vi "BITalino.vi"() -> ()   [LabVIEW 2015]
uses:
  Status.ctl
  Sensor.ctl
  <vilib>/Instr/_visa.llb/VISA Configure Serial Port (Instr).vi
panel:
  in  "DO 4":bool
  in  "DO 3":bool
  in  "DO 2":bool
  in  "DO 1":bool
  in  "Battery \nThreshold (%)":u8(slide)=5 min=5 max=90 step=5 scale=5.0..90.0
  out "CRC Error":bool
  out "tdms file":refnum<k34>
  out "XY Graph":cluster{dbl[], dbl[]}(graph)
  out "Ylabel and Plot name":cluster{string, string}
  out "Sample Rate Numeric":i32
  out "Consumer":i32
  out "producer":i32
  in  "Sensor Selection":enum32{"A1", "A2", "A3", "A4", "A5", "A6"}(radio)
  in  "Sensor 6":T1=enum."LUX"
  in  "Sensor 5":T1=enum."ACC"
  in  "Sensor 4":T1=enum."EDA"
  in  "Sensor 3":T1=enum."EEG"
  in  "Sensor 2":T1=enum."ECG"
  in  "Sensor 1":T1
  out "DI 2":bool
  out "DI 1":bool
  out "DI 4":bool
  out "DI 3":bool
  in  "MODE":bool
  in  "Sample Rate":enum16{"1", "10", "100", "1000"}(ring)=enum."1000"
  in  "error in (no error)":errorcluster
  in  "File Path":path
  in  "X Limit":u32(knob)=5 scale=2.0..30.0
  in  "Device":refnum<visa-resource-name>
  out "Sync Stop":bool=TRUE
  out "Status":T2
  in  "Exit Button":bool
  in  "Record Button":bool
  in  "Stop Button":bool
  # "LIVE MODE"
  # "SIMULATED MODE"
  # "Hz"
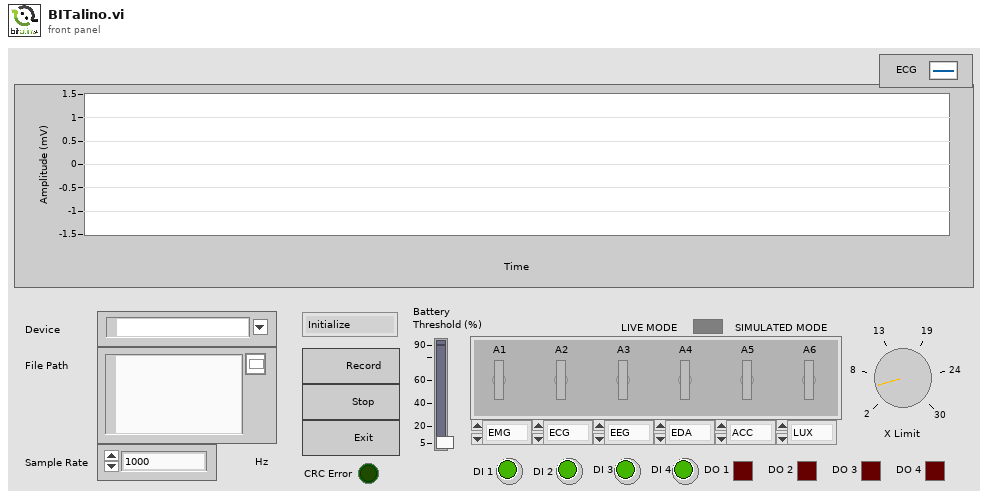
[diagram p1: front panel]
types:
  T1 = typedef "Sensor.ctl" = enum16{"EMG", "ECG", "EEG", "EDA", "ACC", "LUX"}
  T2 = typedef "Status.ctl" = enum16{"Initialize", "Standby", "Recording", "Exit"}
  T3 = enum8{"Enabled", "Disabled", "Disabled and Grayed Out"}
  T4 = enum16{"open", "open or create", "create or replace", "create", "open (read-only)"}
  T5 = cluster{"Sensor 1":T1, "Sensor 2":T1, "Sensor 3":T1, "Sensor 4":T1, "Sensor 5":T1, "Sensor 6":T1}
  T6 = cluster{"Result":dbl, "Result":dbl, "Result":dbl, "Result":dbl, "Result":dbl, "Result":dbl}
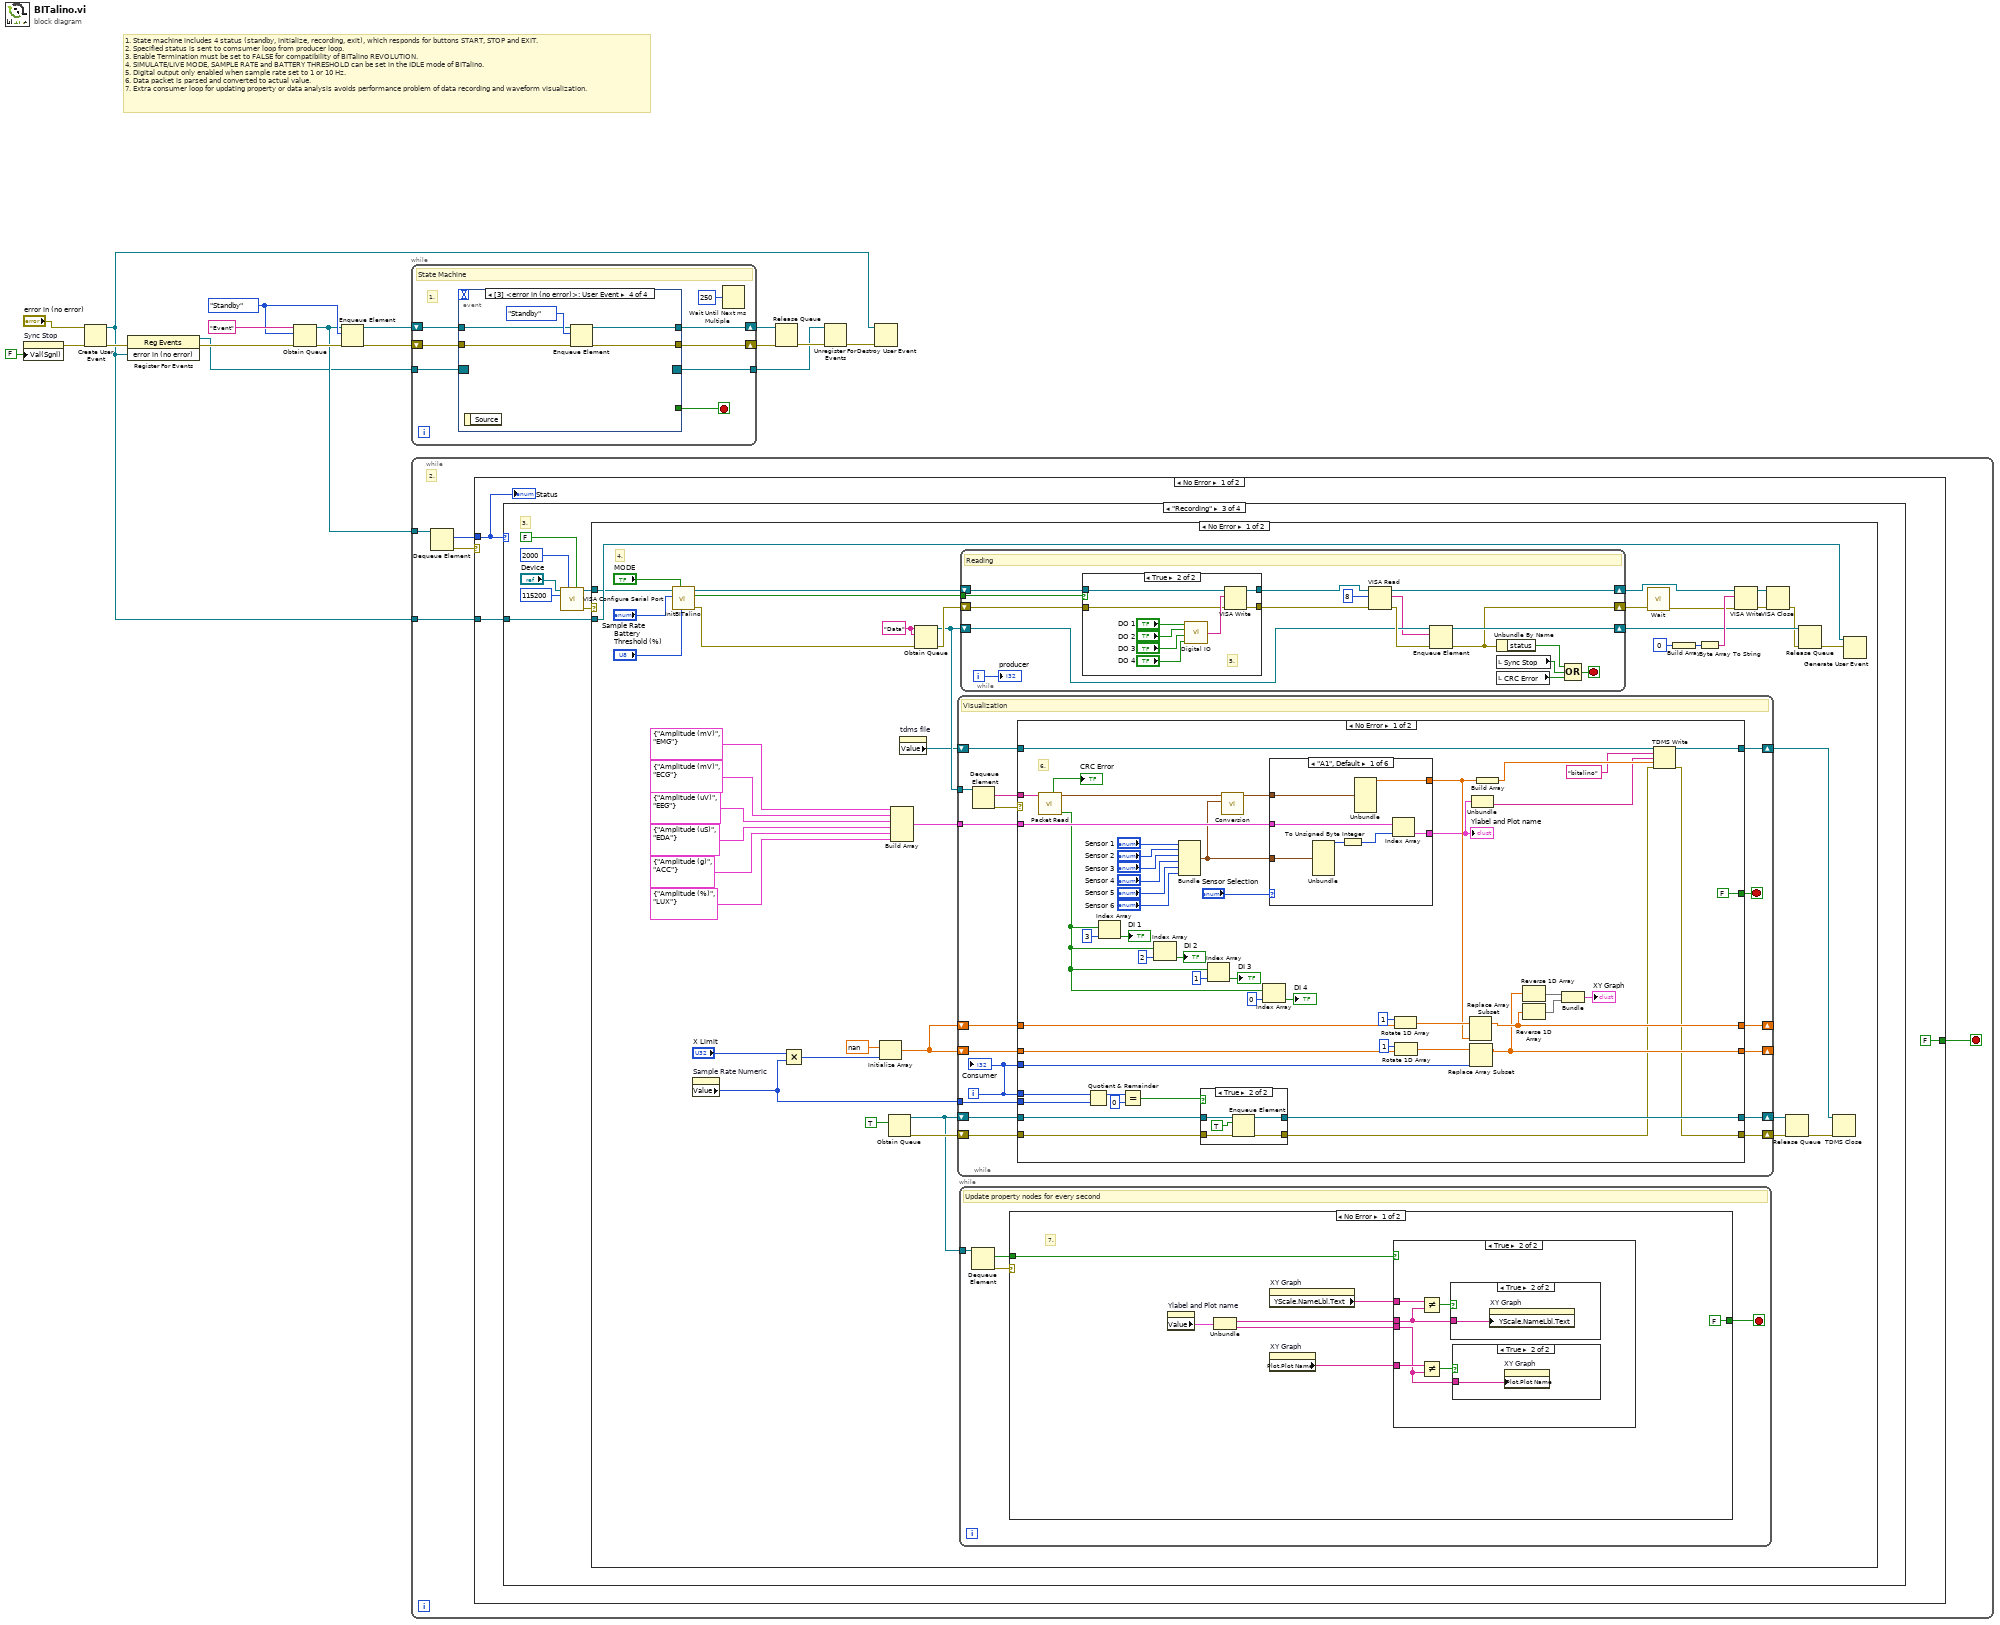
[diagram p0: block diagram]
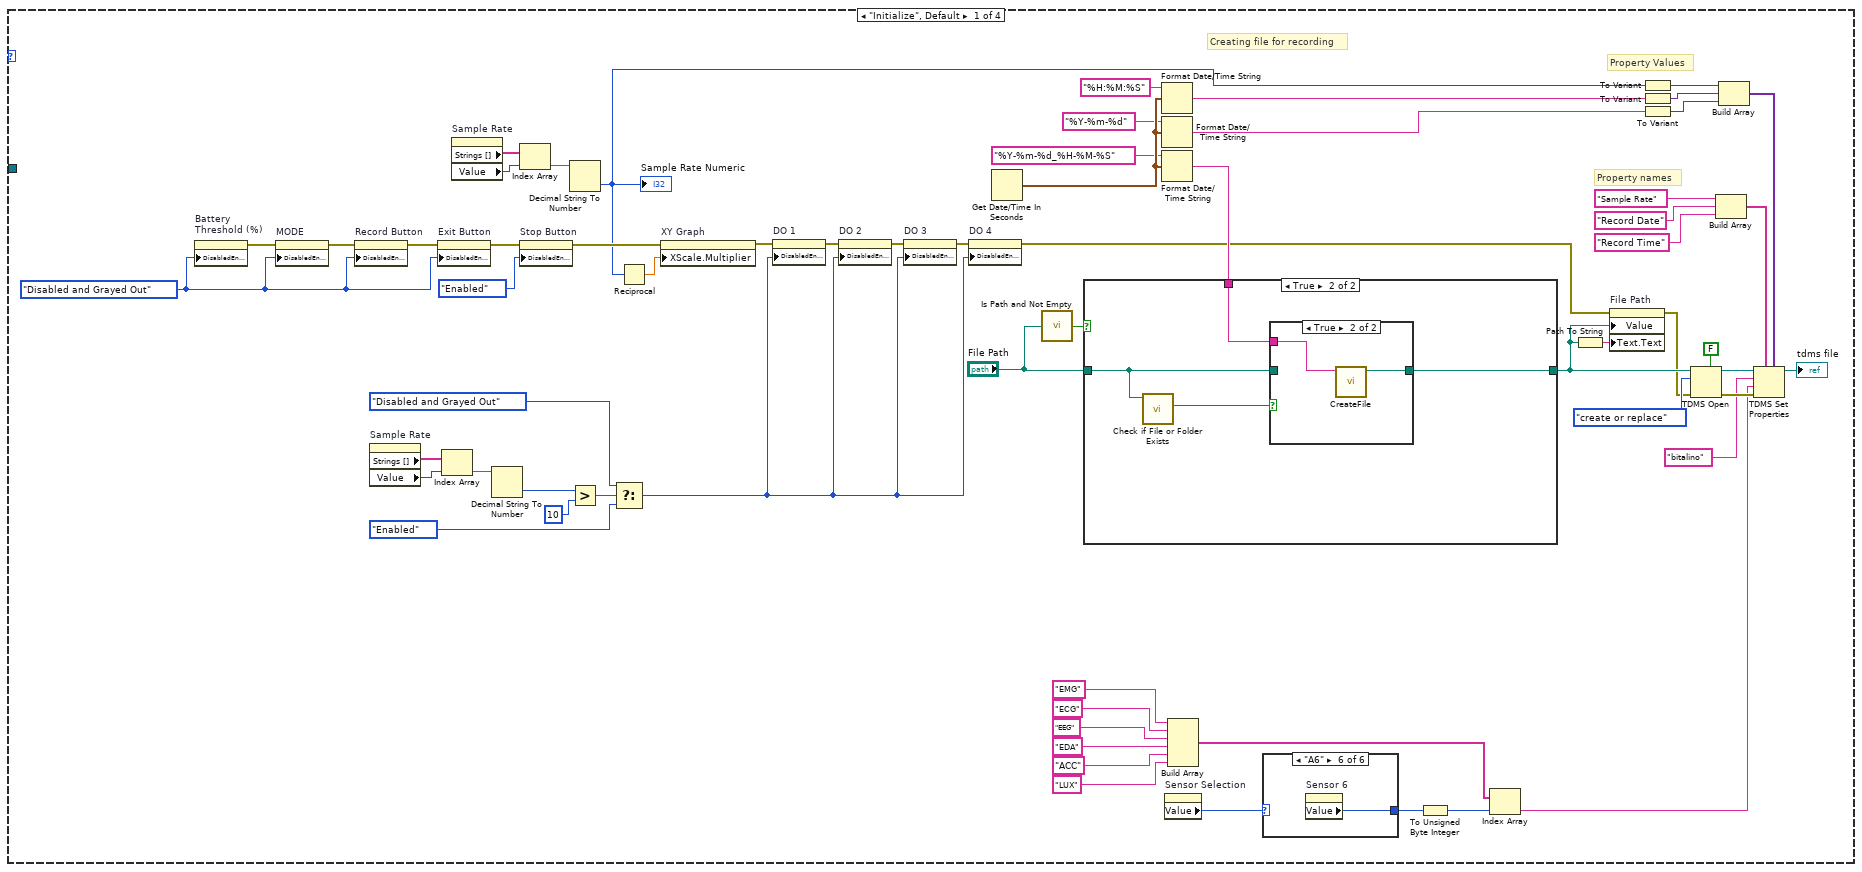
[diagram p2: hidden frame]
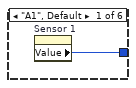
[diagram p3: hidden frame]
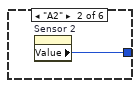
[diagram p4: hidden frame]
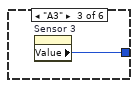
[diagram p5: hidden frame]
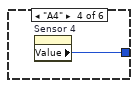
[diagram p6: hidden frame]
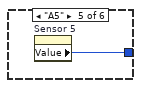
[diagram p7: hidden frame]
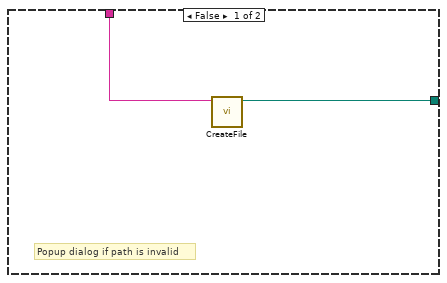
[diagram p8: hidden frame]
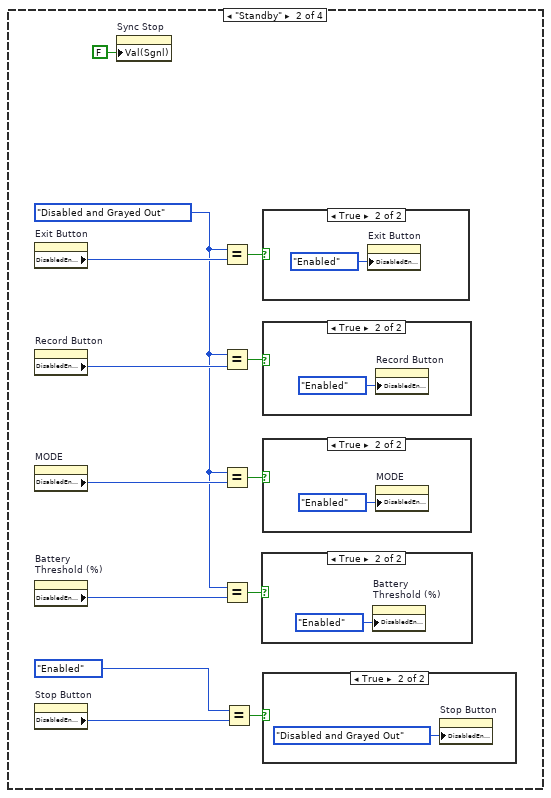
[diagram p10: hidden frame]
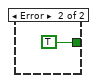
[diagram p19: hidden frame]
diagram:
  w12 = Status."Standby" ("Enum")
  # "1. State machine includes 4 status (standby, initialize, recording, exit), which responds for buttons START, STOP and EXIT.\n2. Specified status is sent to comsumer loop from producer loop.\n3. Enable Termination must be set to FALSE for compatibility of BITalino REVOLUTION.\n4. SIMULATE/LIVE MODE, SAMPLE RATE and BATTERY THRESHOLD can be set in the IDLE mode of BITalino.\n5. Digital output only enabled when sample rate set to 1 or 10 Hz.\n6. Data packet is parsed and converted to actual value.\n7. Extra consumer loop for updating property or data analysis avoids performance problem of data recording and waveform visualization."
  n1 = property on="Sync Stop" class="Bool (strict)"("Val(Sgnl)"=FALSE ("Value (Signaling)")) -> (error out=w9:errorcluster)  [unwired: 2 in, 1 out]
  n2 = Create User Event(user event datatype="error in (no error)", error in=w9) -> (user event=w1:refnum<user-event>, error out=w8:errorcluster)
  n3 = register-events(error in=w8, w1) -> (reference out=w6:refnum<event-registration>, error out=w7:errorcluster)  [unwired: 1 in]
  n4 = Obtain Queue(name (unnamed)="Event", element data type=w12, error in (no error)=w7) -> (queue out=w11:refnum<queue>, error out=w15:errorcluster)  [unwired: 2 in, 1 out]
  n5 = Enqueue Element(queue=w11, element=w12, error in (no error)=w15) -> (queue out=w13:refnum<queue>, error out=w14:errorcluster)  [unwired: 1 in, 1 out]
  n6 = while {
    shift-right: [w23] -> w17
    shift-left: w13 -> [w26]
    shift-right: [w24] -> w16
    shift-left: w14 -> [w25]
    tunnel: w6 -> [w20]
    tunnel: [w19] -> w3
    stop <- w22 stop-if-true
    # "1."
    # "State Machine"
    n7 = event shown="[3] <error in (no error)>: User Event" {
      selector: w20 -> [_ _ _ _]
      dyn-events: [_ _ _ _] -> w19
      timeout: _ -> [_ _ _ _]
      tunnel: w26 -> [w33 w37 w49 w53]
      tunnel: w25 -> [w30 w39 w48 w51]
      tunnel: [w27 w40 w43 w50] -> w24
      tunnel: [w34 w38 w45 w52] -> w23
      tunnel: [FALSE TRUE FALSE _] -> w22
      event "Stop Button": Value Change {
        n8 = event-data() -> ()  [unwired: 1 in, 5 out]
        n9 = Enqueue Element(queue=w33, element=Status."Standby" ("Enum"), error in (no error)=w30) -> (queue out=w34:refnum<queue>, error out=w28:errorcluster)  [unwired: 1 in, 1 out]
        n10 = property on="Sync Stop" class="Bool (strict)"(error in=w28, "Val(Sgnl)"=TRUE) -> (error out=w27:errorcluster)  [unwired: 1 in, 1 out]
      }
      event "Exit Button": Value Change {
        n11 = event-data() -> ()  [unwired: 1 in, 5 out]
        n12 = Enqueue Element(queue=w37, element=Status."Exit" ("Enum"), error in (no error)=w39) -> (queue out=w38:refnum<queue>, error out=w40:errorcluster)  [unwired: 1 in, 1 out]
      }
      event "Record Button": Value Change {
        n13 = event-data() -> ()  [unwired: 1 in, 1 out]
        n14 = Enqueue Element(queue=w49, element=Status."Initialize" ("Enum"), error in (no error)=w48) -> (queue out=w46:refnum<queue>, error out=w44:errorcluster)  [unwired: 1 in, 1 out]
        n15 = Enqueue Element(queue=w46, element=Status."Recording" ("Enum"), error in (no error)=w44) -> (queue out=w45:refnum<queue>, error out=w43:errorcluster)  [unwired: 1 in, 1 out]
      }
      event User Event {
        n16 = event-data() -> ()  [unwired: 1 in, 1 out]
        n17 = Enqueue Element(queue=w53, element=Status."Standby" ("Enum"), error in (no error)=w51) -> (queue out=w52:refnum<queue>, error out=w50:errorcluster)  [unwired: 1 in, 1 out]
      }
    }
    n18 = Wait Until Next ms Multiple(millisecond multiple=u32 250) -> ()  [unwired: 1 out]
  }
  n19 = while {
    tunnel: w11 -> [w58]
    tunnel: w1 -> [w55]
    stop <- w59 stop-if-true
    # "2."
    n20 = Dequeue Element(queue=w58) -> (element=w57:T2, error out=w56:errorcluster)  [unwired: 2 in, 2 out]
    n21 = case shown="No Error" w56 {
      tunnel: w57 -> [w61 _]
      tunnel: [FALSE TRUE] -> w59
      tunnel: w55 -> [w60 _]
      frame No Error {
        n22 = case shown="\"Recording\"" w61 {
          tunnel: w60 -> [_ _ w159 _]
          frame "Initialize", Default {
            w90 = T3."Disabled and Grayed Out" ("Disabled")
            # "Creating file for recording"
            # "Property Values"
            # "Property names"
            n23 = property on="Battery \nThreshold (%)" class="Slide (strict)"("DisabledEnum"=w90) -> (error out=w91:errorcluster)  [unwired: 2 in, 1 out]
            n24 = property on="MODE" class="Bool (strict)"(error in=w91, "DisabledEnum"=w90) -> (error out=w117:errorcluster)  [unwired: 1 in, 1 out]
            n25 = property on="Record Button" class="Bool"(error in=w117, "DisabledEnum"=w90) -> (error out=w125:errorcluster)  [unwired: 1 in, 1 out]
            n26 = property on="Sample Rate" class="Enum (strict)"() -> ("Strings []"=w80:string[], "Value"=w79:enum16{"1", "10", "100", "1000"})  [unwired: 2 in, 2 out]
            n27 = property on="Exit Button" class="Bool"(error in=w125, "DisabledEnum"=w90) -> (error out=w123:errorcluster)  [unwired: 1 in, 1 out]
            n28 = Index Array(array=w80, index=w79) -> (element=w78:string)
            n29 = property on="Sample Rate" class="Enum (strict)"() -> ("Strings []"=w122:string[], "Value"=w121:enum16{"1", "10", "100", "1000"})  [unwired: 2 in, 2 out]
            n30 = Decimal String To Number(string=w78) -> (number=w77:i32)  [unwired: 2 in, 1 out]
            n31 = Index Array(array=w122, index=w121) -> (element=w120:string)
            n32 = property on="Stop Button" class="Bool"(error in=w123, "DisabledEnum"=T3."Enabled" ("Disabled")) -> (error out=w119:errorcluster)  [unwired: 1 in, 1 out]
            n33 = Decimal String To Number(string=w120) -> (number=w89:i32)  [unwired: 2 in, 1 out]
            "Sample Rate Numeric" <- w89
            n34 = Greater?(x=w77, y=10) -> (0:w85:bool)
            n35 = Select(t=T3."Disabled and Grayed Out" ("Disabled"), s=w85, f=T3."Enabled" ("Disabled")) -> (s? t:f=w88:T3)
            n36 = Reciprocal(x=w89) -> (1/x=w118:dbl)
            n37 = property on="XY Graph" class="XYGraph (strict)"(error in=w119, "XScale.Multiplier"=w118) -> (error out=w76:errorcluster)  [unwired: 1 in, 1 out]
            n38 = property on="DO 1" class="Bool (strict)"(error in=w76, "DisabledEnum"=w88) -> (error out=w83:errorcluster)  [unwired: 1 in, 1 out]
            n39 = property on="DO 2" class="Bool (strict)"(error in=w83, "DisabledEnum"=w88) -> (error out=w82:errorcluster)  [unwired: 1 in, 1 out]
            n40 = property on="DO 3" class="Bool (strict)"(error in=w82, "DisabledEnum"=w88) -> (error out=w81:errorcluster)  [unwired: 1 in, 1 out]
            n41 = property on="DO 4" class="Bool (strict)"(error in=w81, "DisabledEnum"=w88) -> (error out=w75:errorcluster)  [unwired: 1 in, 1 out]
            n42 = Get Date/Time In Seconds() -> (seconds since 1Jan1904=w107:timestamp)
            n43 = call <vilib>:"Is Path and Not Empty.vi"("path"="File Path") -> ("Is Path and Not Empty?"=w99:bool)  [unwired: 4 in]
            n44 = Format Date/Time String(time format string (%c)="%H:%M:%S", seconds (now)=w107) -> (date/time string=w112:string)  [unwired: 1 in]
            n45 = Format Date/Time String(time format string (%c)="%Y-%m-%d", seconds (now)=w107) -> (date/time string=w113:string)  [unwired: 1 in]
            n46 = Format Date/Time String(time format string (%c)="%Y-%m-%d_%H-%M-%S", seconds (now)=w107) -> (date/time string=w103:string)  [unwired: 1 in]
            n47 = case shown="True" w99 {
              tunnel: [w132 w135] -> w96
              tunnel: "File Path" -> [_ w134]
              tunnel: w103 -> [w133 w136]
              frame False {
                # "Popup dialog if path is invalid"
                n48 = call "CreateFile.vi"("date/time string"=w133) -> ("appended path"=w132:path)  [unwired: 10 in]
              }
              frame True {
                n49 = call <vilib>:"Check if File or Folder Exists.vi"("path"=w134) -> ("file or folder exists?"=w137:bool)  [unwired: 8 in, 2 out]
                n50 = case shown="True" w137 {
                  tunnel: w136 -> [_ w140]
                  tunnel: [w138 w139] -> w135
                  tunnel: w134 -> [w138 _]
                  frame False {
                  }
                  frame True {
                    n51 = call "CreateFile.vi"("date/time string"=w140) -> ("appended path"=w139:path)  [unwired: 10 in]
                  }
                }
              }
            }
            n52 = property on="Sensor Selection" class="RadioBtnsControl (strict)"() -> ("Value"=w73:enum32{"A1", "A2", "A3", "A4", "A5", "A6"})  [unwired: 2 in, 2 out]
            n53 = Build Array("EMG", "ECG", "EEG", "EDA", "ACC", "LUX") -> (w64:string[])
            n54 = case shown="\"A6\"" w73 {
              tunnel: [w126 w127 w128 w129 w130 w131] -> w66
              frame "A1", Default {
                n55 = property on="Sensor 1" class="Enum (strict)"() -> ("Value"=w126:T1)  [unwired: 2 in, 2 out]
              }
              frame "A2" {
                n56 = property on="Sensor 2" class="Enum (strict)"() -> ("Value"=w127:T1)  [unwired: 2 in, 2 out]
              }
              frame "A3" {
                n57 = property on="Sensor 3" class="Enum (strict)"() -> ("Value"=w128:T1)  [unwired: 2 in, 2 out]
              }
              frame "A4" {
                n58 = property on="Sensor 4" class="Enum (strict)"() -> ("Value"=w129:T1)  [unwired: 2 in, 2 out]
              }
              frame "A5" {
                n59 = property on="Sensor 5" class="Enum (strict)"() -> ("Value"=w130:T1)  [unwired: 2 in, 2 out]
              }
              frame "A6" {
                n60 = property on="Sensor 6" class="Enum (strict)"() -> ("Value"=w131:T1)  [unwired: 2 in, 2 out]
              }
            }
            n61 = To Unsigned Byte Integer(number=w66) -> (unsigned 8bit integer=w65:u8)
            n62 = Index Array(array=w64, index=w65) -> (element=w63:string)
            n63 = Path To String(path=w96) -> (string=w97:string)
            n64 = property on="File Path" class="Path"(error in=w75, "Value"=w96, "Text.Text"=w97) -> (error out=w94:errorcluster)  [unwired: 1 in, 1 out]
            n65 = To Variant(anything=w89) -> (Variant=w111:variant)
            n66 = To Variant(anything=w112) -> (Variant=w114:variant)
            n67 = To Variant(anything=w113) -> (Variant=w115:variant)
            n68 = TDMS Open(5:FALSE ("create index file? (T)"), 8:w94, 10:T4."create or replace" ("operation (0:open)"), 11:w96) -> (0:w102:errorcluster, 3:w101:refnum<k34>)  [unwired: 3 in]
            n69 = Build Array("Sample Rate", "Record Date", "Record Time") -> (w110:string[])
            n70 = Build Array(w111, w114, w115) -> (w116:variant[])
            n71 = TDMS Set Properties(5:w116, 7:w110, 8:w102, 9:w63, 10:"bitalino", 11:w101) -> (3:→"tdms file":refnum<k34>)  [unwired: 3 out]
          }
          frame "Standby" {
            w141 = T3."Disabled and Grayed Out" ("Disabled")
            n72 = property on="Exit Button" class="Bool"() -> ("DisabledEnum"=w152:T3)  [unwired: 2 in, 2 out]
            n73 = property on="Record Button" class="Bool"() -> ("DisabledEnum"=w150:T3)  [unwired: 2 in, 2 out]
            n74 = property on="MODE" class="Bool (strict)"() -> ("DisabledEnum"=w144:T3)  [unwired: 2 in, 2 out]
            n75 = property on="Battery \nThreshold (%)" class="Slide (strict)"() -> ("DisabledEnum"=w142:T3)  [unwired: 2 in, 2 out]
            n76 = property on="Stop Button" class="Bool"() -> ("DisabledEnum"=w147:T3)  [unwired: 2 in, 2 out]
            n77 = property on="Sync Stop" class="Bool (strict)"("Val(Sgnl)"=FALSE ("Value (Signaling)")) -> ()  [unwired: 2 in, 2 out]
            n78 = Equal?(x=w141, y=w152) -> (x = y?=w151:bool)
            n79 = Equal?(x=w141, y=w150) -> (x = y?=w149:bool)
            n80 = Equal?(x=w141, y=w144) -> (x = y?=w145:bool)
            n81 = Equal?(x=w141, y=w142) -> (x = y?=w143:bool)
            n82 = Equal?(x=T3."Enabled" ("Disabled"), y=w147) -> (x = y?=w146:bool)
            n83 = case shown="True" w143 {
              frame False {
              }
              frame True {
                n84 = property on="Battery \nThreshold (%)" class="Slide (strict)"("DisabledEnum"=T3."Enabled" ("Disabled")) -> ()  [unwired: 2 in, 2 out]
              }
            }
            n85 = case shown="True" w151 {
              frame False {
              }
              frame True {
                n86 = property on="Exit Button" class="Bool"("DisabledEnum"=T3."Enabled" ("Disabled")) -> ()  [unwired: 2 in, 2 out]
              }
            }
            n87 = case shown="True" w149 {
              frame False {
              }
              frame True {
                n88 = property on="Record Button" class="Bool"("DisabledEnum"=T3."Enabled" ("Disabled")) -> ()  [unwired: 2 in, 2 out]
              }
            }
            n89 = case shown="True" w145 {
              frame False {
              }
              frame True {
                n90 = property on="MODE" class="Bool (strict)"("DisabledEnum"=T3."Enabled" ("Disabled")) -> ()  [unwired: 2 in, 2 out]
              }
            }
            n91 = case shown="True" w146 {
              frame False {
              }
              frame True {
                n92 = property on="Stop Button" class="Bool"("DisabledEnum"=T3."Disabled and Grayed Out" ("Disabled")) -> ()  [unwired: 2 in, 2 out]
              }
            }
          }
          frame "Recording" {
            # "3."
            n93 = call-poly "VISA Configure Serial Port"("VISA resource name"="Device", "timeout (10sec)"=u32 2000, "Enable Termination\nChar (T)"=FALSE ("Enable Termination\nChar (T)"), "baud rate (9600)"=u32 115200) -> ("VISA resource name out"=w162:refnum<visa-resource-name>, "error out"=w161:errorcluster)  [unwired: 10 in]
            n94 = case shown="No Error" w161 {
              selector: w161 -> [_ w380]
              tunnel: w162 -> [w192 _]
              tunnel: w159 -> [w194 w381]
              frame No Error {
                w202 = "Data"
                # "4."
                n95 = call "InitBITalino.vi"("Battery \nThreshold (%)"="Battery \nThreshold (%)", "MODE"="MODE", "Sample Rate"="Sample Rate", "BITalino"=w192) -> ("error out"=w166:errorcluster, "Digital Output"=w167:bool, "VISA out"=w169:refnum<visa-resource-name>)  [unwired: 5 in]
                n96 = property on="Sample Rate Numeric" class="DigNum (strict)"() -> ("Value"=w183:i32)  [unwired: 2 in, 2 out]
                n97 = Multiply(x="X Limit", y=w183) -> (x*y=w181:u32)
                n98 = Initialize Array(nan ("element"), w181) -> (w180:dbl[])
                n99 = Obtain Queue(element data type=TRUE) -> (queue out=w186:refnum<queue>, error out=w188:errorcluster)  [unwired: 4 in, 1 out]
                n100 = Build Array(cluster{string, string} {"Amplitude (mV)", "EMG"}, cluster{string, string} {"Amplitude (mV)", "ECG"}, cluster{string, string} {"Amplitude (uV)", "EEG"}, cluster{string, string} {"Amplitude (uS)", "EDA"}, cluster{string, string} {"Amplitude (g)", "ACC"}, cluster{string, string} {"Amplitude (%)", "LUX"}) -> (w173:cluster{string, string}[])
                n101 = property on="tdms file" class="Ref (strict)"() -> ("Value"=w172:refnum<k34>)  [unwired: 2 in, 2 out]
                n102 = Obtain Queue(name (unnamed)=w202, element data type=w202, error in (no error)=w166) -> (queue out=w203:refnum<queue>, error out=w204:errorcluster)  [unwired: 2 in, 1 out]
                n103 = while {
                  tunnel: w203 -> [w244]
                  shift-right: [w239] -> _
                  shift-left: w180 -> [w240]
                  tunnel: w183 -> [w238]
                  shift-right: [w235] -> w185
                  shift-left: w186 -> [w237]
                  shift-right: [w234] -> w184
                  shift-left: w188 -> [w236]
                  shift-right: [w231] -> _
                  shift-left: w180 -> [w233]
                  tunnel: w173 -> [w230]
                  shift-right: [w228] -> w170
                  shift-left: w172 -> [w229]
                  i -> [w232]
                  stop <- w242 stop-if-true
                  # "Visualization"
                  n104 = Dequeue Element(queue=w244) -> (element=w241:string, error out=w243:errorcluster)  [unwired: 2 in, 2 out]
                  n105 = case shown="No Error" w243 {
                    tunnel: [FALSE TRUE] -> w242
                    tunnel: w241 -> [w259 _]
                    tunnel: w240 -> [w280 w350]
                    tunnel: [w276 w350] -> w239
                    tunnel: w238 -> [w281 _]
                    tunnel: w232 -> [w286 _]
                    tunnel: w237 -> [w289 w349]
                    tunnel: w236 -> [w288 w348]
                    tunnel: [w287 w349] -> w235
                    tunnel: [w261 w348] -> w234
                    tunnel: w233 -> [w277 w347]
                    tunnel: w232 -> [w271 _]
                    tunnel: [w275 w347] -> w231
                    tunnel: w230 -> [w270 _]
                    tunnel: w229 -> [w266 w346]
                    tunnel: [w265 w346] -> w228
                    frame No Error {
                      # "6."
                      n106 = call "Packet Read.vi"("Packets"=w259) -> ("Digital IO"=w250:bool[], "Analog Channels"=w258:cluster{u16, u16, u16, u16, u16, u16}, "CRC Error"=→"CRC Error":bool)  [unwired: 7 in, 1 out]
                      n107 = Quotient & Remainder(x=w286, y=w281) -> (x-y*floor(x/y)=w285:i32)  [unwired: 1 out]
                      n108 = Index Array(array=w250, index=3) -> (element=→"DI 1":bool)
                      n109 = Equal?(x=w285, y=0) -> (x = y?=w283:bool)
                      n110 = Index Array(array=w250, index=2) -> (element=→"DI 2":bool)
                      n111 = Bundle("Sensor 1"="Sensor 1", "Sensor 2"="Sensor 2", "Sensor 3"="Sensor 3", "Sensor 4"="Sensor 4", "Sensor 5"="Sensor 5", "Sensor 6"="Sensor 6") -> (w269:T5)  [unwired: 1 in]
                      n112 = case shown="True" w283 {
                        tunnel: w289 -> [w298 w303]
                        tunnel: w288 -> [w297 w302]
                        tunnel: [w298 w301] -> w287
                        tunnel: [w297 w300] -> w264
                        frame False {
                        }
                        frame True {
                          n113 = Enqueue Element(queue=w303, element=TRUE, error in (no error)=w302) -> (queue out=w301:refnum<queue>, error out=w300:errorcluster)  [unwired: 1 in, 1 out]
                        }
                      }
                      n114 = Index Array(array=w250, index=1) -> (element=→"DI 3":bool)
                      n115 = call "Conversion.vi"("Sensor Type"=w269, "Analog Channels"=w258) -> ("Converted Values"=w291:T6)  [unwired: 8 in, 1 out]
                      n116 = Index Array(array=w250, index=0) -> (element=→"DI 4":bool)
                      n117 = case shown="\"A1\", Default" "Sensor Selection" {
                        tunnel: w291 -> [w310 w317 w324 w331 w338 w345]
                        tunnel: [w309 w316 w323 w330 w337 w344] -> w263
                        tunnel: w270 -> [w305 w312 w319 w327 w333 w341]
                        tunnel: w269 -> [w308 w314 w321 w328 w335 w342]
                        tunnel: [w304 w311 w320 w326 w334 w340] -> w247
                        frame "A1", Default {
                          n118 = Unbundle(w308) -> ("Sensor 1"=w306:T1)  [unwired: 5 out]
                          n119 = To Unsigned Byte Integer(number=w306) -> (unsigned 8bit integer=w307:u8)
                          n120 = Unbundle(w310) -> ("Result"=w309:dbl)  [unwired: 5 out]
                          n121 = Index Array(array=w305, index=w307) -> (element=w304:cluster{string, string})
                        }
                        frame "A2" {
                          n122 = Unbundle(w314) -> ("Sensor 2"=w313:T1)  [unwired: 5 out]
                          n123 = To Unsigned Byte Integer(number=w313) -> (unsigned 8bit integer=w315:u8)
                          n124 = Unbundle(w317) -> ("Result"=w316:dbl)  [unwired: 5 out]
                          n125 = Index Array(array=w312, index=w315) -> (element=w311:cluster{string, string})
                        }
                        frame "A3" {
                          n126 = Unbundle(w321) -> ("Sensor 3"=w318:T1)  [unwired: 5 out]
                          n127 = To Unsigned Byte Integer(number=w318) -> (unsigned 8bit integer=w322:u8)
                          n128 = Unbundle(w324) -> ("Result"=w323:dbl)  [unwired: 5 out]
                          n129 = Index Array(array=w319, index=w322) -> (element=w320:cluster{string, string})
                        }
                        frame "A4" {
                          n130 = Unbundle(w328) -> ("Sensor 4"=w325:T1)  [unwired: 5 out]
                          n131 = To Unsigned Byte Integer(number=w325) -> (unsigned 8bit integer=w329:u8)
                          n132 = Unbundle(w331) -> ("Result"=w330:dbl)  [unwired: 5 out]
                          n133 = Index Array(array=w327, index=w329) -> (element=w326:cluster{string, string})
                        }
                        frame "A5" {
                          n134 = Unbundle(w335) -> ("Sensor 5"=w332:T1)  [unwired: 5 out]
                          n135 = Unbundle(w338) -> ("Result"=w337:dbl)  [unwired: 5 out]
                          n136 = To Unsigned Byte Integer(number=w332) -> (unsigned 8bit integer=w336:u8)
                          n137 = Index Array(array=w333, index=w336) -> (element=w334:cluster{string, string})
                        }
                        frame "A6" {
                          n138 = Unbundle(w342) -> ("Sensor 6"=w339:T1)  [unwired: 5 out]
                          n139 = To Unsigned Byte Integer(number=w339) -> (unsigned 8bit integer=w343:u8)
                          n140 = Unbundle(w345) -> ("Result"=w344:dbl)  [unwired: 5 out]
                          n141 = Index Array(array=w341, index=w343) -> (element=w340:cluster{string, string})
                        }
                      }
                      "Ylabel and Plot name" <- w247
                      n142 = Rotate 1D Array(1:w280, 2:1 ("n")) -> (0:w282:dbl[])
                      n143 = Rotate 1D Array(1:w277, 2:1 ("n")) -> (0:w278:dbl[])
                      n144 = Replace Array Subset(array=w282, new element=w263) -> (w276:dbl[])  [unwired: 1 in]
                      n145 = Replace Array Subset(array=w278, new element=w271) -> (w275:dbl[])  [unwired: 1 in]
                      n146 = Unbundle(w247) -> (w246:string)  [unwired: 1 out]
                      n147 = Build Array(w263) -> (w262:dbl[])
                      n148 = Reverse 1D Array(array=w275) -> (reversed array=w274:dbl[])
                      n149 = Reverse 1D Array(array=w276) -> (reversed array=w273:dbl[])
                      n150 = Bundle(w274, w273) -> (→"XY Graph":cluster{dbl[], dbl[]})  [unwired: 1 in]
                      n151 = TDMS Write(0:w266, 5:"bitalino", 7:w246, 9:w262, 11:w264) -> (4:w265:refnum<k34>, 15:w261:errorcluster)  [unwired: 1 in, 2 out]
                    }
                    frame Error {
                    }
                  }
                  "Consumer" <- w232
                }
                n152 = while {
                  tunnel: w186 -> [w211]
                  stop <- w208 stop-if-true
                  # "Update property nodes for every second"
                  n153 = Dequeue Element(queue=w211) -> (element=w209:bool, error out=w210:errorcluster)  [unwired: 2 in, 2 out]
                  n154 = case shown="No Error" w210 {
                    tunnel: w209 -> [w215 _]
                    tunnel: [FALSE TRUE] -> w208
                    frame No Error {
                      # "7."
                      n155 = property on="Ylabel and Plot name" class="Clust (strict)"() -> ("Value"=w218:cluster{string, string})  [unwired: 2 in, 2 out]
                      n156 = Unbundle(w218) -> (w217:string, w216:string)
                      n157 = property on="XY Graph" class="XYGraph (strict)"() -> ("YScale.NameLbl.Text"=w213:string)  [unwired: 2 in, 2 out]
                      n158 = property on="XY Graph" class="XYGraph (strict)"() -> ("Plot.Plot Name"=w212:string)  [unwired: 2 in, 2 out]
                      n159 = case shown="True" w215 {
                        tunnel: w213 -> [_ w224]
                        tunnel: w212 -> [_ w220]
                        tunnel: w217 -> [_ w221]
                        tunnel: w216 -> [_ w219]
                        frame False {
                        }
                        frame True {
                          n160 = Not Equal?(x=w224, y=w221) -> (x != y?=w222:bool)
                          n161 = Not Equal?(x=w220, y=w219) -> (x != y?=w223:bool)
                          n162 = case shown="True" w222 {
                            tunnel: w221 -> [_ w226]
                            frame False {
                            }
                            frame True {
                              n163 = property on="XY Graph" class="XYGraph (strict)"("YScale.NameLbl.Text"=w226) -> ()  [unwired: 2 in, 2 out]
                            }
                          }
                          n164 = case shown="True" w223 {
                            tunnel: w219 -> [_ w225]
                            frame False {
                            }
                            frame True {
                              n165 = property on="XY Graph" class="XYGraph (strict)"("Plot.Plot Name"=w225) -> ()  [unwired: 2 in, 2 out]
                            }
                          }
                        }
                      }
                    }
                    frame Error {
                    }
                  }
                }
                n166 = while {
                  shift-right: [w365] -> w198
                  shift-left: w204 -> [w355]
                  shift-right: [w366] -> w201
                  shift-left: w203 -> [w367]
                  shift-right: [w364] -> w200
                  shift-left: w169 -> [w354]
                  tunnel: w167 -> [w352]
                  i -> [w361]
                  stop <- w360 stop-if-true
                  # "Reading"
                  n167 = case shown="True" w352 {
                    tunnel: [w370 w379] -> w356
                    tunnel: w355 -> [w369 w373]
                    tunnel: w354 -> [w370 w372]
                    tunnel: [w369 w371] -> w353
                    frame False {
                    }
                    frame True {
                      # "5."
                      n168 = call "Digital IO.vi"("DO 4"="DO 4", "DO 3"="DO 3", "DO in"="DO 2", "DO 1"="DO 1") -> ("string"=w378:string)
                      n169 = VISA Write(VISA resource name=w372, write buffer=w378, error in (no error)=w373) -> (VISA resource name out=w379:refnum<visa-resource-name>, error out=w371:errorcluster)  [unwired: 1 out]
                    }
                  }
                  n170 = VISA Read(VISA resource name=w356, byte count=u32 8, error in (no error)=w353) -> (VISA resource name out=w364:refnum<visa-resource-name>, read buffer=w363:string, error out=w368:errorcluster)  [unwired: 1 out]
                  n171 = Enqueue Element(queue=w367, element=w363, error in (no error)=w368) -> (queue out=w366:refnum<queue>, error out=w365:errorcluster)  [unwired: 1 in, 1 out]
                  n172 = Unbundle By Name(w365) -> ("status"=w358:bool)
                  n173 = local read "Sync Stop"() -> (w359:bool)
                  n174 = local read "CRC Error"() -> (w357:bool)
                  n175 = Compound Arithmetic op=OR(w358, w359, w357) -> (w360:bool)
                  "producer" <- w361
                }
                n176 = call "Wait.vi"("error in (no error)"=w198) -> ("error out"=w199:errorcluster)  [unwired: 10 in]
                n177 = Build Array(u8 0) -> (w206:u8[])
                n178 = Byte Array To String(unsigned byte array=w206) -> (string=w205:string)
                n179 = VISA Write(VISA resource name=w200, write buffer=w205, error in (no error)=w199) -> (VISA resource name out=w196:refnum<visa-resource-name>, error out=w197:errorcluster)  [unwired: 1 out]
                n180 = VISA Close(VISA resource name=w196, error in (no error)=w197) -> (error out=w195:errorcluster)
                n181 = Release Queue(queue=w185, error in (no error)=w184) -> (error out=w171:errorcluster)  [unwired: 1 in, 2 out]
                n182 = Release Queue(queue=w201, error in (no error)=w195) -> (error out=w193:errorcluster)  [unwired: 1 in, 2 out]
                n183 = TDMS Close(8:w171, 11:w170) -> ()  [unwired: 2 out]
                n184 = Generate User Event(user event=w194, event data cluster=w193) -> ()  [unwired: 2 in, 2 out]
              }
              frame Error {
                n185 = Generate User Event(user event=w381, event data cluster=w380) -> ()  [unwired: 2 in, 2 out]
              }
            }
          }
          frame "Exit" {
            n186 = flat-sequence {
              frame #0 {
                n187 = property on="Stop Button" class="Bool"("DisabledEnum"=T3."Enabled" ("Disabled")) -> ()  [unwired: 2 in, 2 out]
              }
              frame #1 {
                n188 = Stop(stop? (T)=TRUE) -> ()
              }
            }
          }
        }
        "Status" <- w61
      }
      frame Error {
      }
    }
  }
  n189 = Release Queue(queue=w17, error in (no error)=w16) -> (error out=w4:errorcluster)  [unwired: 1 in, 2 out]
  n190 = Unregister For Events(event registration refnum=w3, error in=w4) -> (error out=w2:errorcluster)
  n191 = Destroy User Event(user event=w1, error in=w2) -> ()  [unwired: 1 out]
